vi "computeDisplayImages.vi"() -> ()   [LabVIEW 2017]
uses:
  <vilib>/Analysis/baseanly.llb/Std Deviation and Variance.vi
  globalUtilities.vi
  globalDevices.vi
panel:
  in  "axis":u16(ring) items=["x", "y", "z"]
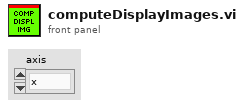
[diagram p1: front panel]
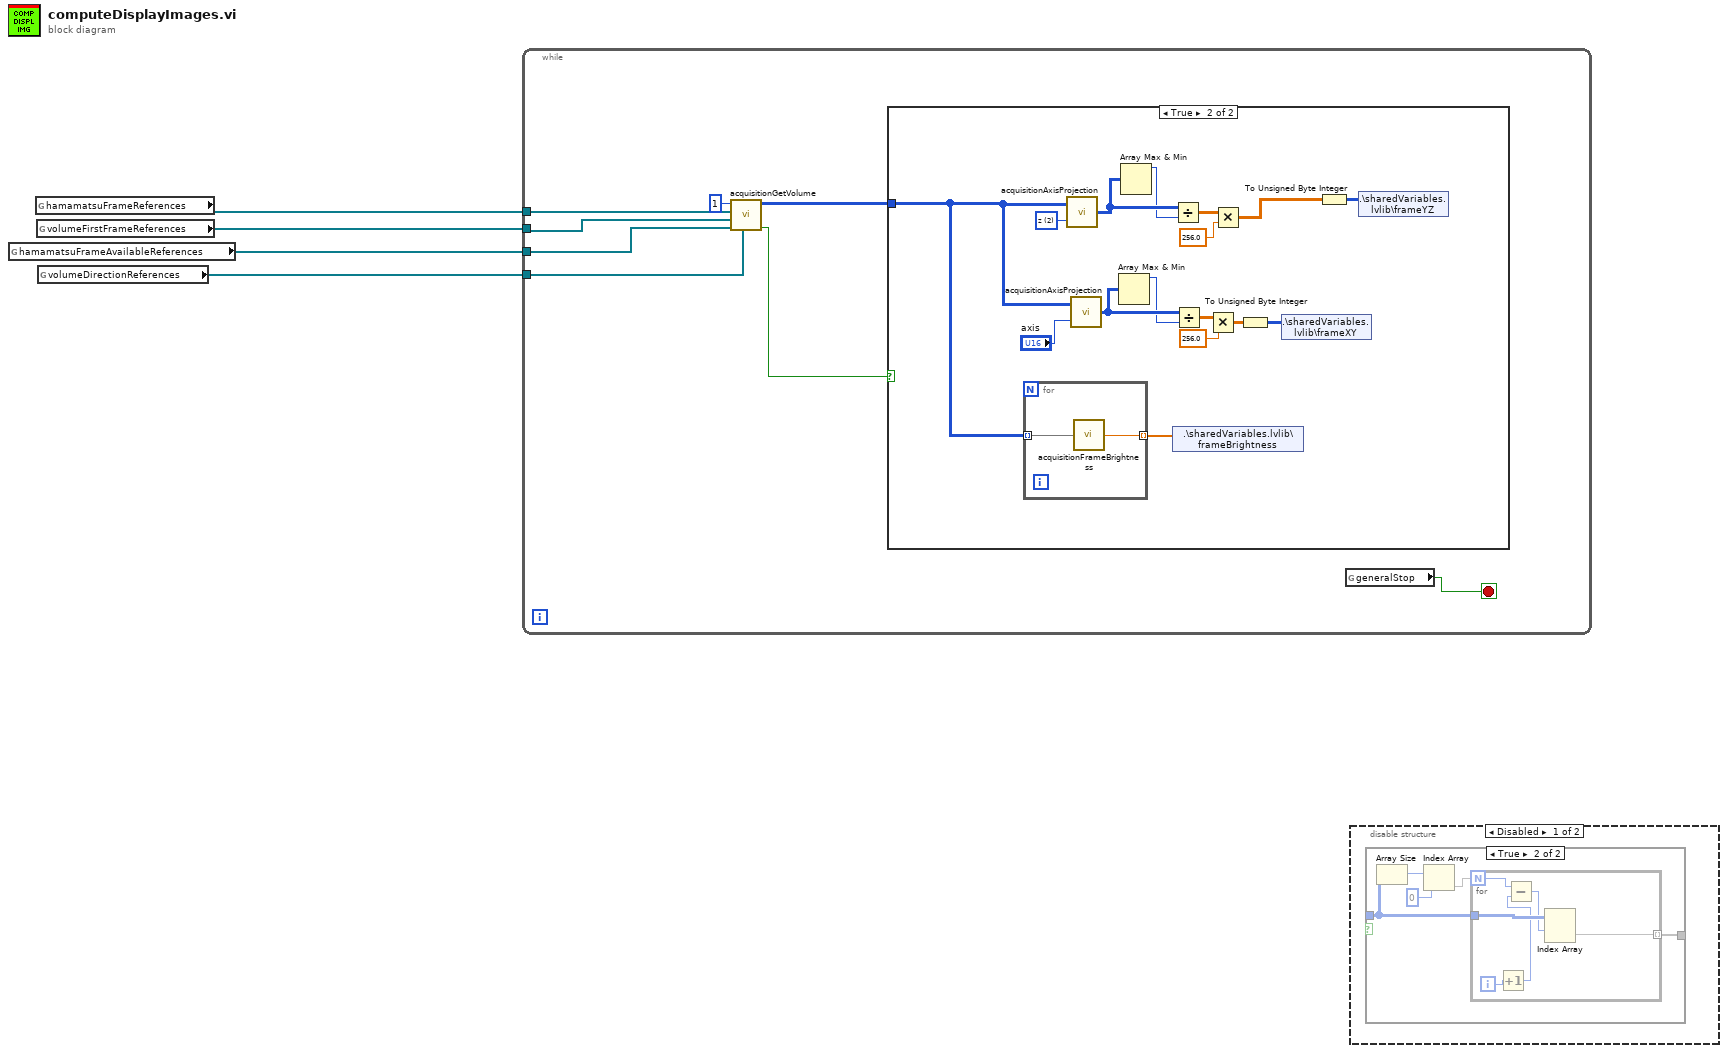
[diagram p0: block diagram]
diagram:
  n1 = global read "globalDevices.vi" "hamamatsuFrameAvailableReferences"() -> (w3:refnum<data-value>[])
  n2 = global read "globalDevices.vi" "hamamatsuFrameReferences"() -> (w4:refnum<data-value>[])
  n3 = global read "globalUtilities.vi" "volumeFirstFrameReferences"() -> (w2:refnum<data-value>[])
  n4 = global read "globalUtilities.vi" "volumeDirectionReferences"() -> (w1:refnum<data-value>[])
  n5 = while {
    tunnel: w4 -> [w12]
    tunnel: w3 -> [w11]
    tunnel: w2 -> [w7]
    tunnel: w1 -> [w6]
    stop <- w8 stop-if-true
    n6 = call "acquisitionGetVolume.vi"("volumeDirectionReferences"=w6, "hamamatsuFrameAvailableReferences"=w11, "volumeFirstFrameReferences"=w7, "hamamatsuFrameReferences"=w12, "volume index (last: 0)"=1) -> ("success"=w9:bool, "volume out"=w10:u16[][][])  [unwired: 3 out]
    n7 = case shown="True" w9 {
      tunnel: w10 -> [_ w14]
      frame False {
      }
      frame True {
        w28 = u16 2 items=["x", "y", "z"] ("axis (z)")
        n8 = for {
          tunnel: w14 -> [w30] mode=indexing
          tunnel: [w29] -> w13 mode=indexing
          n9 = call "acquisitionFrameBrightness.vi"("frame"=w30) -> ("brighness"=w29:dbl)
        }
        n10 = call "acquisitionAxisProjection.vi"("axis (z)"=w28, "z stack"=w14) -> ("projected img"=w26:u64[][])
        n11 = call "acquisitionAxisProjection.vi"("axis (z)"="axis", "z stack"=w14) -> ("projected img"=w21:u64[][])
        n12 = Array Max & Min(array=w21) -> (max value=w20:u64)  [unwired: 3 out]
        n13 = Array Max & Min(array=w26) -> (max value=w25:u64)  [unwired: 3 out]
        n14 = Divide(x=w26, y=w25) -> (x/y=w24:dbl[][])
        n15 = shared-variable ".\\sharedVariables.lvlib\\frameBrightness"(w13) -> ()  [unwired: 1 in, 1 out]
        n16 = Divide(x=w21, y=w20) -> (x/y=w19:dbl[][])
        n17 = Multiply(x=w19, y=256.0) -> (x*y=w17:dbl[][])
        n18 = Multiply(x=w24, y=256.0) -> (x*y=w22:dbl[][])
        n19 = To Unsigned Byte Integer(number=w17) -> (unsigned 8bit integer=w16:u8[][])
        n20 = shared-variable ".\\sharedVariables.lvlib\\frameXY"(w16) -> ()  [unwired: 1 in, 1 out]
        n21 = To Unsigned Byte Integer(number=w22) -> (unsigned 8bit integer=w15:u8[][])
        n22 = shared-variable ".\\sharedVariables.lvlib\\frameYZ"(w15) -> ()  [unwired: 1 in, 1 out]
      }
    }
    n23 = global read "globalUtilities.vi" "generalStop"() -> (w8:bool)
  }
  n24 = disable-structure shown="Disabled" {
    frame Disabled {
      n25 = case shown="True" {
        selector: _ -> [_ _]
        tunnel: _ -> [w31 w36]
        tunnel: [w31 w32] -> _
        frame False {
        }
        frame True {
          n26 = Array Size(array=w36) -> (size(s)=w35:i32)
          n27 = Index Array(array=w35, index=0) -> (element=w33)
          n28 = for {
            N: w33 -> [w41]
            tunnel: w36 -> [w42]
            tunnel: [w37] -> w32 mode=indexing
            i -> [w40]
            n29 = Increment(x=w40) -> (x+1=w39:i32)
            n30 = Subtract(x=w41, y=w39) -> (x-y=w38:i32)
            n31 = Index Array(array=w42, index (row)=w38) -> (element=w37)  [unwired: 1 in]
          }
        }
      }
    }
    frame Enabled {
    }
  }
